vi "JTAG_Cyclone_SoftFP.vi"(0 "reference in":refnum<class "JTAG_Cyclone.lvclass">, 2 "Floating":bool, 5 "error in (no error)":errorcluster) -> (14 "reference out":refnum<class "JTAG_Cyclone.lvclass">, 19 "error out":errorcluster)   [LabVIEW 2022 SP3, in "JTAG_Cyclone.lvlib" / "JTAG_Cyclone.lvclass"]
uses:
  JTAG_Cyclone.lvclass
  Components/ViPER.lvlibp/ViPER.lvclass
  C:/Projects/Medulla/Presentations/Sydney_LVUG/Demo/Flux_Capacitor_Tester/Components/ViPER.lvlibp/ViPER.lvclass
panel:
  in  "Image":string
  out "Success":bool
  out "Msg":string
  in  "Program":bool
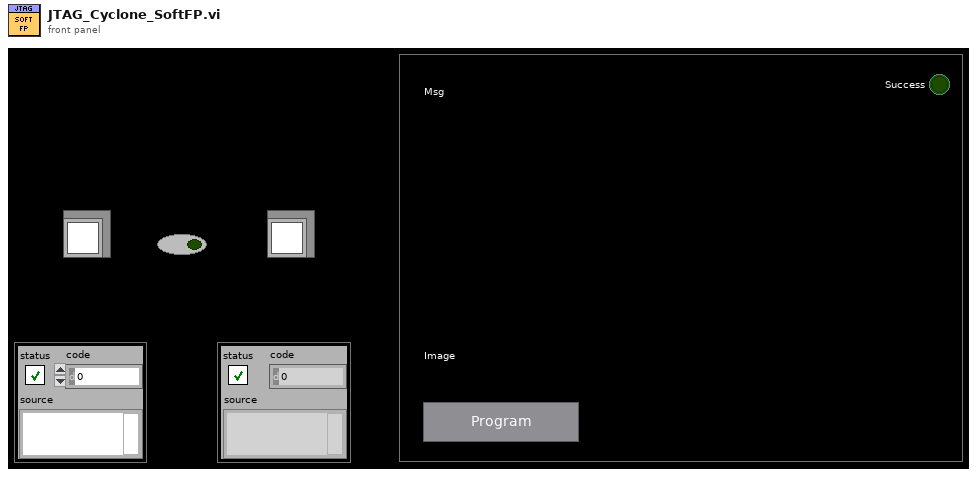
[diagram p1: front panel]
types:
  T1 = enum32{"Invalid", "Standard", "Closed", "Hidden", "Minimized", "Maximized"}
  T2 = typedef "JTAG_Cyclone.lvlib/JTAG_Cyclone.lvclass/ObjectAttributes.ctl" = cluster{"Config":T3, "Success":bool, "Msg":string, "active image":string}
  T3 = typedef "JTAG_Cyclone.lvlib/JTAG_Cyclone.lvclass/Config.ctl" = cluster{"Cyclone_API_Path":path, "Cyclone_Name":string}
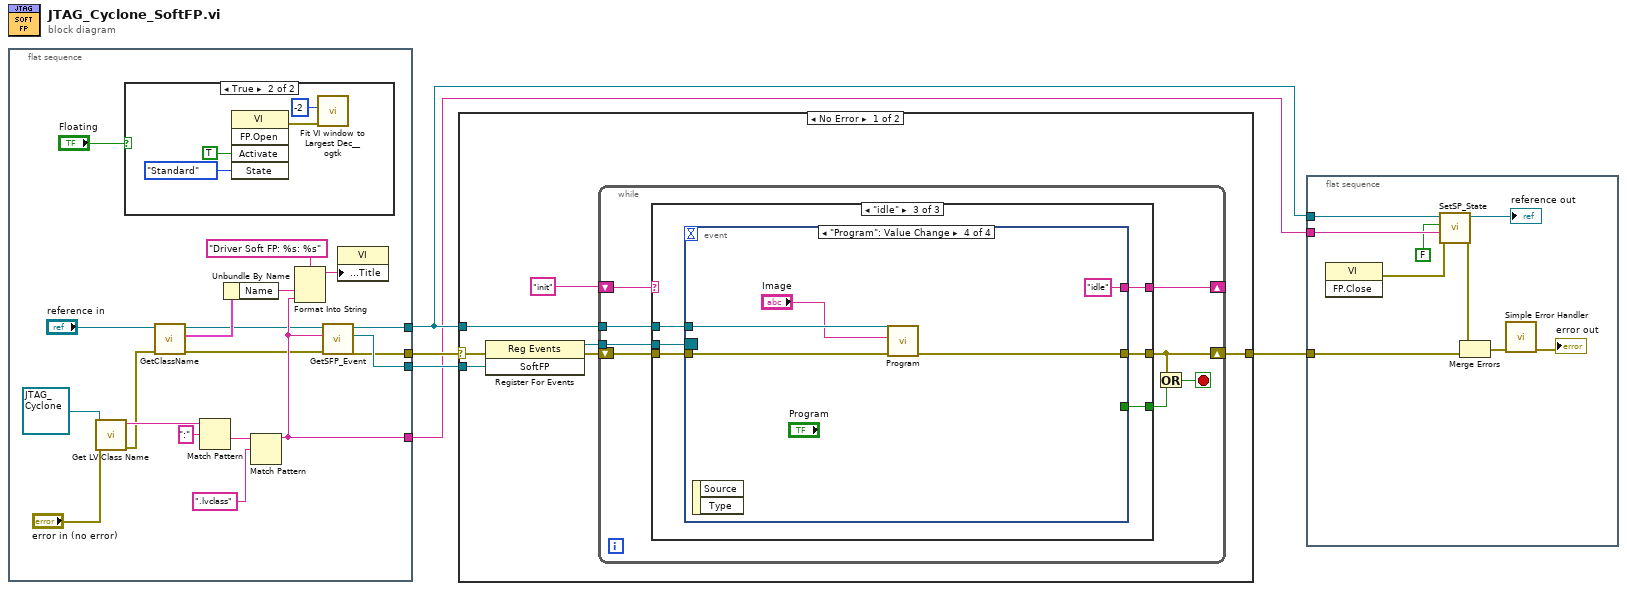
[diagram p0: block diagram]
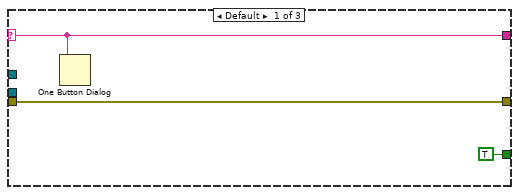
[diagram p3: hidden frame]
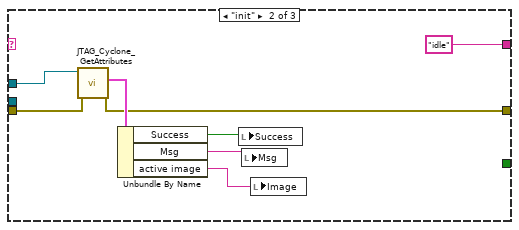
[diagram p4: hidden frame]
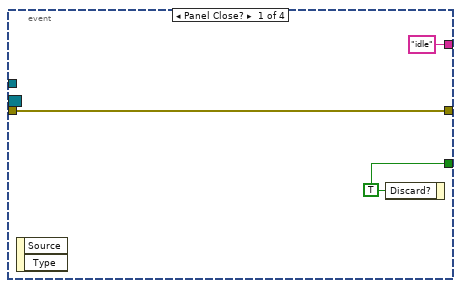
[diagram p5: hidden frame]
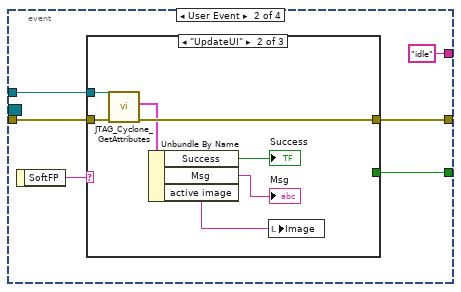
[diagram p6: hidden frame]
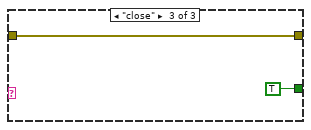
[diagram p8: hidden frame]
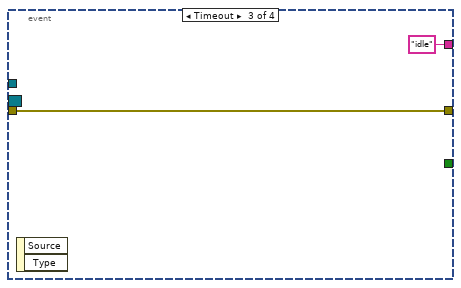
[diagram p9: hidden frame]
diagram:
  n1 = flat-sequence {
    tunnel: [w21] -> w5
    tunnel: [w20] -> w2
    tunnel: [w24] -> w3
    tunnel: [w12] -> w1
    frame #0 {
      n2 = call <vilib>:"Get LV Class Name.vi"("error in (no error)"="error in (no error)", "object"=refnum<class "JTAG_Cyclone.lvclass"> refnum ("reference")) -> ("error out"=w11:errorcluster, "class name"=w17:string)  [unwired: 8 in]
      n3 = case shown="True" "Floating" {
        frame False {
        }
        frame True {
          n4 = invoke class="VI" method="FP.Open"("Activate"=TRUE ("Activate?"), "State"=T1."Standard") -> (error out=w25:errorcluster)  [unwired: 3 in, 4 out]
          n5 = call <userlib>:"Fit VI window to Largest Dec__ogtk.vi"("error in (no error)"=w25, "border spacing (2 px)"=-2) -> ()  [unwired: 4 in, 2 out]
        }
      }
      n6 = call "GetClassName.vi"("error in (no error)"=w11, "reference in"="reference in") -> ("error out"=w10:errorcluster, "Details"=w9:cluster{"Name":string, "Class":string}, "reference out"=w7:refnum<class "JTAG_Cyclone.lvclass">)  [unwired: 7 in]
      n7 = Match Pattern(string=w17, regular expression=":") -> (after substring=w15:string)  [unwired: 1 in, 3 out]
      n8 = Unbundle By Name(w9) -> ("Name"=w19:string)
      n9 = Match Pattern(string=w15, regular expression=".lvclass") -> (before substring=w12:string)  [unwired: 1 in, 3 out]
      n10 = Format Into String(format string="Driver Soft FP: %s: %s", w19, w12) -> (resulting string=w23:string)  [unwired: 2 in, 1 out]
      n11 = call-dynamic "GetSFP_Event.vi"("error in (no error)"=w10, "Ancestor"=w12, "reference in"=w7) -> ("error out"=w21:errorcluster, "SoftFP"=w24:refnum<user-event>, "reference out"=w20:refnum<class "JTAG_Cyclone.lvclass">)  [unwired: 6 in]
      n12 = property class="VI"("Front Panel.Title"=w23) -> ()  [unwired: 2 in, 2 out]
    }
  }
  n13 = case shown="No Error" w5 {
    selector: w5 -> [w33 w87]
    tunnel: [w29 w87] -> w4
    tunnel: w2 -> [w30 _]
    tunnel: w3 -> [w35 _]
    frame No Error {
      n14 = register-events(error in=w33, w35) -> (reference out=w34:refnum<event-registration>, error out=w32:errorcluster)  [unwired: 1 in]
      n15 = while {
        shift-right: [w40] -> w29
        shift-left: w32 -> [w43]
        tunnel: w34 -> [w42]
        tunnel: w30 -> [w41]
        shift-right: [w36] -> _
        shift-left: "init" -> [w37]
        stop <- w39 stop-if-true
        n16 = case shown="\"idle\"" w37 {
          selector: w37 -> [w44 _ _]
          tunnel: w43 -> [w45 w51 w60]
          tunnel: w42 -> [_ _ w59]
          tunnel: w41 -> [_ w52 w58]
          tunnel: [w45 w50 w57] -> w40
          tunnel: [TRUE ("Discard?") _ w56] -> w38
          tunnel: [w44 "idle" w55] -> w36
          frame Default {
            n17 = One Button Dialog(message=w44) -> ()  [unwired: 1 in, 1 out]
          }
          frame "init" {
            n18 = call "JTAG_Cyclone_GetAttributes.vi"("error in (no error)"=w51, "reference in"=w52) -> ("error out"=w50:errorcluster, "Data"=w53:T2)  [unwired: 6 in, 2 out]
            n19 = Unbundle By Name(w53) -> ("Success"=w48:bool, "Msg"=w49:string, "active image"=w47:string)
            n20 = local write "Success"(w48) -> ()
            n21 = local write "Msg"(w49) -> ()
            n22 = local write "Image"(w47) -> ()
          }
          frame "idle" {
            n23 = event shown="[3] \"Program\": Value Change" {
              selector: w59 -> [_ _ _ _]
              dyn-events: _ -> [_ _ _ _]
              timeout: _ -> [_ _ _ _]
              tunnel: w60 -> [w63 w69 w81 w85]
              tunnel: [w63 w67 w81 w84] -> w57
              tunnel: [w62 w66 _ _] -> w56
              tunnel: w58 -> [_ w64 _ w83]
              tunnel: ["idle" "idle" "idle" "idle"] -> w55
              event Panel Close? {
                w62 = TRUE ("Discard?")
                n24 = event-data() -> ()  [unwired: 1 in, 2 out]
                n25 = event-data("Discard?"=w62) -> ()  [unwired: 1 in, 1 out]
              }
              event User Event {
                n26 = event-data() -> ("SoftFP"=w68:string)  [unwired: 1 in]
                n27 = case shown="\"UpdateUI\"" w68 {
                  tunnel: w69 -> [w70 w77 w79]
                  tunnel: [w70 w75 w79] -> w67
                  tunnel: [_ _ TRUE ("Discard?")] -> w66
                  tunnel: w64 -> [_ w76 _]
                  frame Default {
                  }
                  frame "UpdateUI" {
                    n28 = call "JTAG_Cyclone_GetAttributes.vi"("error in (no error)"=w77, "reference in"=w76) -> ("error out"=w75:errorcluster, "Data"=w74:T2)  [unwired: 6 in, 2 out]
                    n29 = Unbundle By Name(w74) -> ("Success"=→"Success":bool, "Msg"=→"Msg":string, "active image"=w71:string)
                    n30 = local write "Image"(w71) -> ()
                  }
                  frame "close" {
                  }
                }
              }
              event Timeout {
                n31 = event-data() -> ()  [unwired: 1 in, 2 out]
              }
              event "Program": Value Change {
                n32 = event-data() -> ()  [unwired: 1 in, 2 out]
                n33 = call-dynamic "Program.vi"("error in (no error)"=w85, "Image"="Image", "reference in"=w83) -> ("error out"=w84:errorcluster)  [unwired: 5 in, 3 out]
              }
            }
          }
        }
        n34 = Or(x=w40, y=w38) -> (x .or. y?=w39:bool)
      }
    }
    frame Error {
    }
  }
  n35 = flat-sequence {
    tunnel: w4 -> [w94]
    tunnel: w2 -> [w89]
    tunnel: w1 -> [w91]
    frame #0 {
      n36 = invoke class="VI" method="FP.Close"() -> (error out=w93:errorcluster)  [unwired: 3 in, 2 out]
      n37 = call "SetSP_State.vi"("error in (no error)"=w93, "Ancestor"=w91, "SP Open"=FALSE, "reference in"=w89) -> ("error out"=w92:errorcluster, "reference out"=→"reference out":refnum<class "JTAG_Cyclone.lvclass">)  [unwired: 6 in]
      n38 = Merge Errors(w92, w94) -> (w96:errorcluster)
      n39 = call <vilib>:"Simple Error Handler.vi"("error in (no error)"=w96) -> ("error out"=→"error out":errorcluster)  [unwired: 4 in, 4 out]
    }
  }
